vi "tdms.is_valid_channel.vi"(10 "TDMS Property Names":string[](array[string])) -> (2 "Valid Channel":bool)   [LabVIEW 2019, in "Nominal Client.lvclass"]
doc: "A TDMS channel is valid if it contains waveform data (wf_increment, wf_start_time)."
uses:
  Nominal Client.lvclass
  Nominal Client.lvclass/Nominal Client.ctl
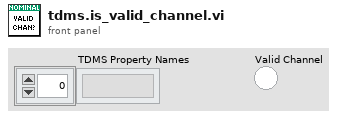
[diagram p1: front panel]
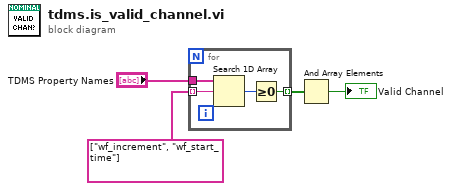
[diagram p0: block diagram]
diagram:
  n1 = for {
    tunnel: "TDMS Property Names" -> [w8]
    tunnel: string[] ["wf_increment", "wf_start_time"] ("element") -> [w7] mode=indexing
    tunnel: [w5] -> w3 mode=indexing
    n2 = Search 1D Array(1D array=w8, element=w7) -> (index of element=w6:i32)  [unwired: 1 in]
    n3 = Greater Or Equal To 0?(x=w6) -> (x >= 0?=w5:bool)
  }
  n4 = And Array Elements(Boolean array=w3) -> (logical AND=→"Valid Channel":bool)
